vi "SEQ.vi"(8 "error in (no error)":errorcluster) -> (0 "error out":errorcluster, 1 "Created New?":bool, 3 "Modules":refnum<queue>)   [LabVIEW 2022 SP3, in "Core.lvlib" / "Module.lvlib"]
uses:
  Module.lvlib
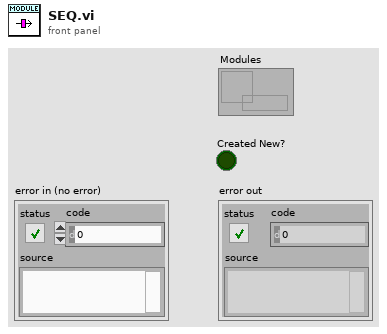
[diagram p1: front panel]
types:
  T1 = cluster{"ID":i32, "Name":string, "Parent ID":i32, "Instance":refnum<data-value>}[]
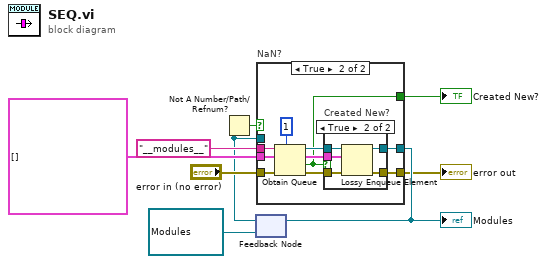
[diagram p0: block diagram]
diagram:
  n1 = feedback #1(refnum<queue> refnum ("queue out")) -> (w4:refnum<queue>)
  n2 = Not A Number/Path/Refnum?(number/path/refnum=w4) -> (NaN/Path/Refnum?=w3:bool)
  n3 = case "NaN?" shown="True" w3 {
    tunnel: T1 [] ("Modules") -> [_ w16]
    tunnel: "__modules__" ("name (unnamed)") -> [_ w20]
    tunnel: [w11 w17] -> w7
    tunnel: "error in (no error)" -> [w10 w14]
    tunnel: [w10 w13] -> w5
    tunnel: w4 -> [w11 _]
    tunnel: [_ w12] -> w1
    frame False {
    }
    frame True {
      n4 = Obtain Queue(max queue size (-1, unlimited)=1, name (unnamed)=w20, element data type=w16, error in (no error)=w14) -> (queue out=w18:refnum<queue>, created new?=w12:bool, error out=w15:errorcluster)  [unwired: 1 in]
      n5 = case "Created New?" shown="True" w12 {
        tunnel: w18 -> [w22 w27]
        tunnel: [w22 w26] -> w17
        tunnel: w16 -> [_ w25]
        tunnel: w15 -> [w21 w24]
        tunnel: [w21 w23] -> w13
        frame False {
        }
        frame True {
          n6 = Lossy Enqueue Element(queue=w27, element=w25, error in (no error)=w24) -> (queue out=w26:refnum<queue>, error out=w23:errorcluster)  [unwired: 2 out]
        }
      }
    }
  }
  "error out" <- w5
  "Modules" <- w7
  "Created New?" <- w1
  n7 = feedback-in #1(w7) -> ()
